vi "Untitled 1.vi"() -> ()   [LabVIEW 2014]
uses:
  <vilib>/Utility/miscctls.llb/LVBoundsTypeDef.ctl
  WNCPacking/system/FunctionFolder/RobotContrl/Global/PCTRL_LinkData.vi
panel:
  in  "stop":bool
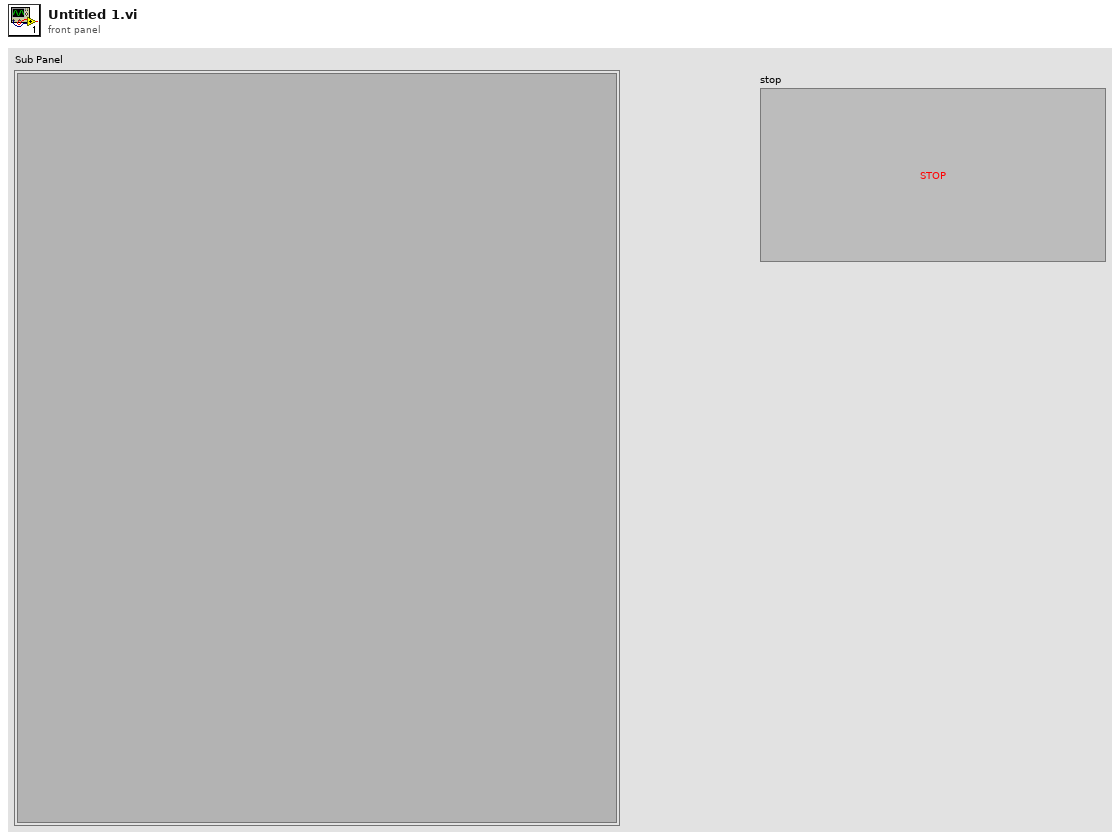
[diagram p1: front panel]
types:
  T1 = typedef "LVBoundsTypeDef.ctl" = cluster{"Width":u32, "Height":u32}
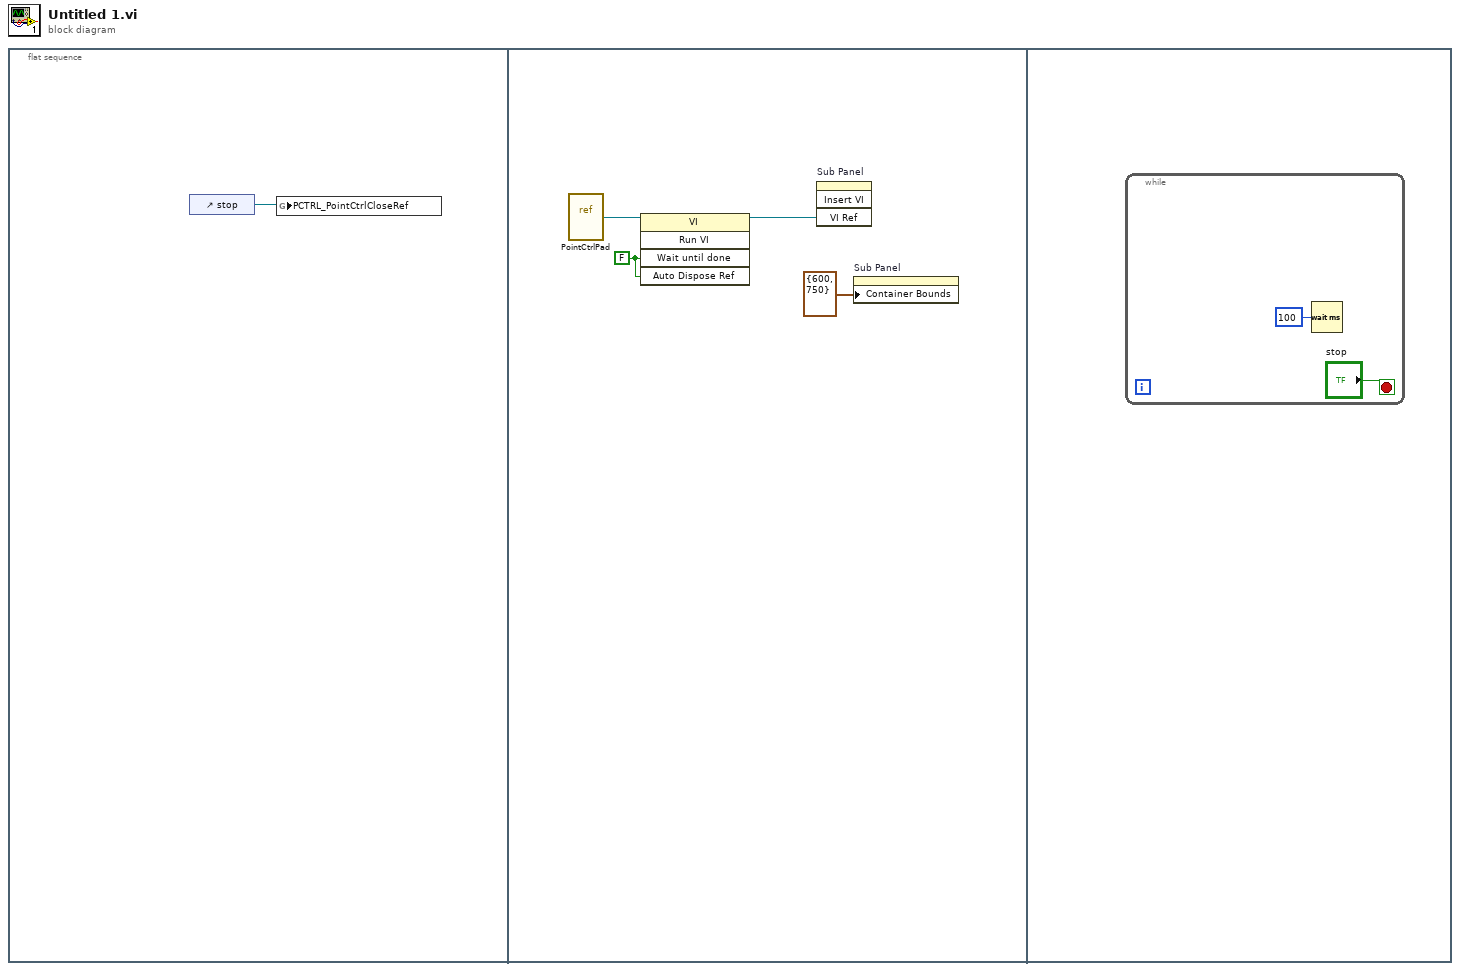
[diagram p0: block diagram]
diagram:
  n1 = flat-sequence {
    frame #0 {
      n2 = control-ref of="stop"() -> (w1:refnum<vi>)
      n3 = global write "PCTRL_LinkData.vi" "PCTRL_PointCtrlCloseRef"(w1) -> ()
    }
    frame #1 {
      w4 = FALSE ("Wait Until Done")
      n4 = vi-ref "PointCtrlPad.vi"() -> (w5:refnum<vi>)
      n5 = invoke class="VI" method="Run VI"(reference=w5, "Wait until done"=w4, "Auto Dispose Ref"=w4) -> (reference out=w3:refnum<vi>)  [unwired: 2 in, 4 out]
      n6 = invoke on="Sub Panel" class="SubPnl" method="Insert VI"("VI Ref"=w3) -> ()  [unwired: 3 in, 4 out]
      n7 = property on="Sub Panel" class="SubPnl"("Container Bounds"=T1 {"Width"=600, "Height"=750}) -> ()  [unwired: 2 in, 2 out]
    }
    frame #2 {
      n8 = while {
        stop <- "stop" stop-if-true
        n9 = Wait (ms)(milliseconds to wait=u32 100) -> ()  [unwired: 1 out]
      }
    }
  }
